vi "Call Scheduler LUT.vi"(7 "command":T2=enum."calculate times", 8 "error in":errorcluster, 9 "pending frames":u32[](array[numeric]), 10 "frame schedule":T1 {"Arb ID" format="%.0x"}, 11 "scheduler lut":T3) -> (0 "error out":errorcluster, 1 "frames to generate":u32[](array[numeric]))   [LabVIEW 2013, in "J1939.lvlib"]
uses:
  J1939.lvlib
  Cyclic Frame Scheduler Lut Reference.ctl
  Cyclic Frame Scheduler LUT Command.ctl
  API Types/Periodic Message Generator Cluster.ctl
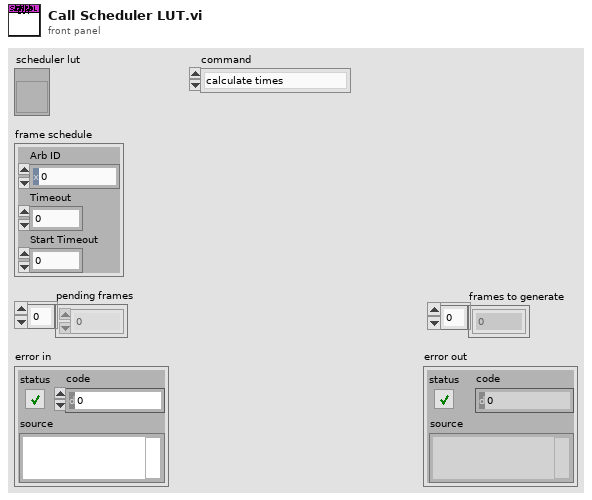
[diagram p1: front panel]
types:
  T1 = typedef "J1939.lvlib/Periodic Message Generator Cluster.ctl" = cluster{"Arb ID":u32, "Timeout":u32, "Start Timeout":u32}
  T2 = typedef "J1939.lvlib/cyclic frame scheduler lut command.ctl" = enum16{"Initialize", "set", "remove", "calculate times"}
  T3 = typedef "J1939.lvlib/cyclic frame scheduler lut reference.ctl" = refnum<vi>
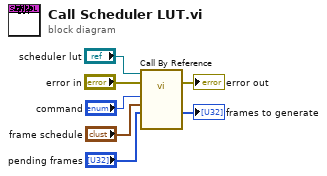
[diagram p0: block diagram]
diagram:
  n1 = call-by-ref "?"(reference="scheduler lut", error in="error in", "pending frames"="pending frames", "frame schedule"="frame schedule", "command"="command") -> (error out=→"error out":errorcluster, "frames to generate"=→"frames to generate":u32[])  [unwired: 8 in, 1 out]
